vi "ErrorCodes.vi"(8 "error in (no error)":errorcluster) -> (0 "error out":errorcluster, 3 "description":string)   [LabVIEW 2021]
uses:
  <vilib>/Utility/error.llb/DialogType.ctl
  <vilib>/Utility/error.llb/Error Cluster From Error Code.vi
  <vilib>/ErrorRing/Error Ring.xnode
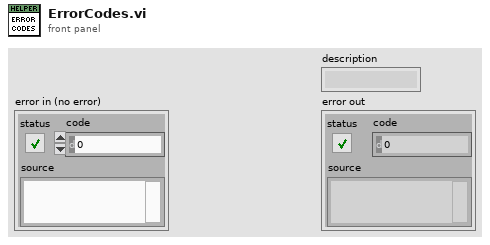
[diagram p1: front panel]
types:
  T1 = typedef "DialogType.ctl" = u16
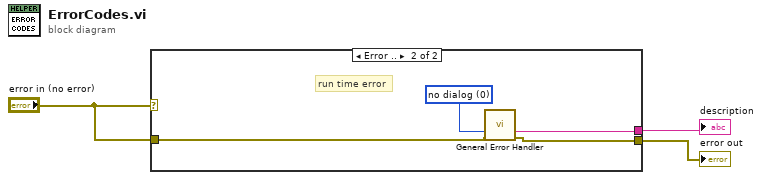
[diagram p0: block diagram]
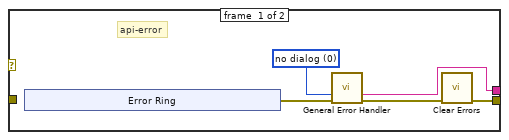
[diagram p2: hidden frame]
diagram:
  n1 = case shown="Error .." "error in (no error)" {
    tunnel: "error in (no error)" -> [_ w17]
    tunnel: [w7 w14] -> w3
    tunnel: [w4 w15] -> w2
    frame #0 {
      w5 = T1 0 items=["no dialog", "OK message", "continue or stop message", "OK message + warnings", "continue/stop + warnings"] ("type of dialog (OK msg:1)")
      # "api-error"
      n2 = xnode "Error Ring"() -> ("error out"=w8:errorcluster)
      n3 = call <vilib>:"General Error Handler.vi"("type of dialog (OK msg:1)"=w5, "error in (no error)"=w8) -> ("message"=w7:string, "error out"=w6:errorcluster)  [unwired: 9 in, 3 out]
      n4 = call <vilib>:"Clear Errors.vi"("error in (no error)"=w6) -> ("error out"=w4:errorcluster)  [unwired: 5 in, 1 out]
    }
    frame #1 {
      w16 = T1 0 items=["no dialog", "OK message", "continue or stop message", "OK message + warnings", "continue/stop + warnings"] ("type of dialog (OK msg:1)")
      # "run time error"
      n5 = call <vilib>:"General Error Handler.vi"("type of dialog (OK msg:1)"=w16, "error in (no error)"=w17) -> ("message"=w14:string, "error out"=w15:errorcluster)  [unwired: 9 in, 3 out]
    }
  }
  "description" <- w3
  "error out" <- w2
